vi "Do.vi"(8 "error in (no error)":errorcluster, 10 "Actor in":refnum<class "Actor.lvclass">, 11 "StartMeasurement":refnum<class "StartMeasurement_Msg.lvclass">) -> (0 "error out":errorcluster, 2 "Actor out":refnum<class "Actor.lvclass">)   [LabVIEW 2010, in "Actor1_GUI_N_4.0.0.lvlib" / "StartMeasurement_Msg.lvclass"]
doc: "(<B>Filename</B>: Actor Framework.lvlib:Message.lvclass:Do.vi)\n\nDefines what a message does when it is received by an actor. Generally, a message instructs an actor to invoke one of its methods.\n\nBy default, this method does nothing. A child class must override it to define behavior. Create a child class by using the Actor Framework Message Maker dialog box."
uses:
  StartMeasurement_Msg.lvclass
  <vilib>/ActorFramework/Actor/Actor.lvclass
  Actor1_GUI_N_4.0.0_class/Actor1_GUI_N_4.0.0.lvclass
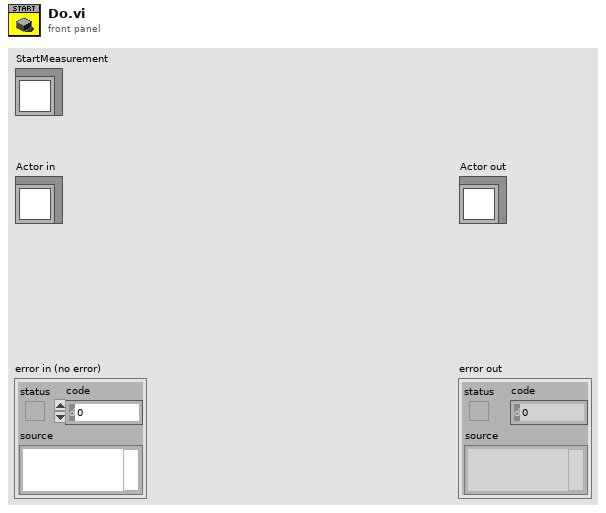
[diagram p1: front panel]
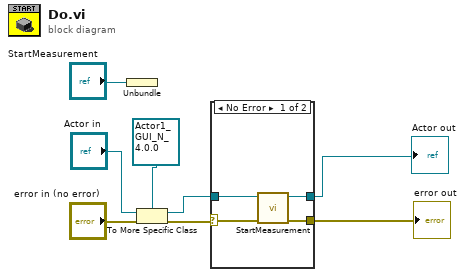
[diagram p0: block diagram]
diagram:
  n1 = Unbundle("StartMeasurement") -> ()  [unwired: 1 out]
  n2 = To More Specific Class(target class=refnum<class "Actor1_GUI_N_4.0.0.lvclass"> refnum ("object in"), reference="Actor in", error in="error in (no error)") -> (specific class reference=w5:refnum<class "Actor1_GUI_N_4.0.0.lvclass">, error out=w3:errorcluster)
  n3 = case shown="No Error" w3 {
    selector: w3 -> [w10 w14]
    tunnel: w5 -> [w12 w13]
    tunnel: [w11 w13] -> w4
    tunnel: [w9 w14] -> w2
    frame No Error {
      n4 = call-dynamic "StartMeasurement.vi"("error in (no error)"=w10, "object in"=w12) -> ("error out"=w9:errorcluster, "object out"=w11:refnum<class "Actor1_GUI_N_4.0.0.lvclass">)  [unwired: 8 in]
    }
    frame Error {
    }
  }
  "error out" <- w2
  "Actor out" <- w4
